vi "first_enable.vi"(2 "error out 2":errorcluster, 3 "VISA resource name 2":refnum<visa-resource-name>) -> (0 "error out 3":errorcluster, 1 "VISA resource name 3":refnum<visa-resource-name>)   [LabVIEW 2017]
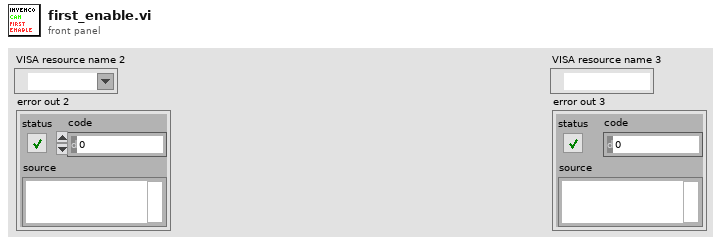
[diagram p1: front panel]
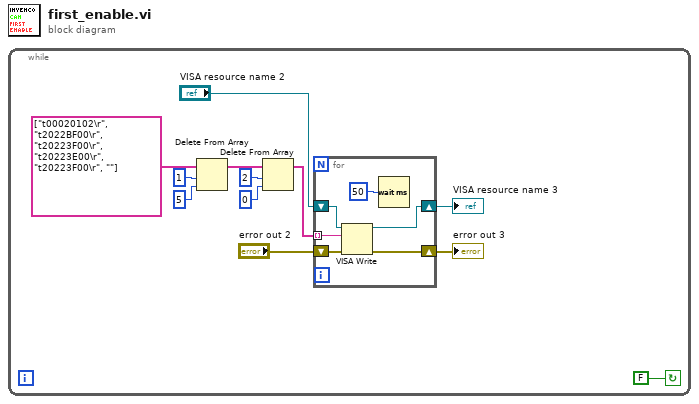
[diagram p0: block diagram]
diagram:
  n1 = while {
    stop <- FALSE continue-if-true
    n2 = Delete From Array(array=string[] ["t00020102\r", "t2022BF00\r", "t20223F00\r", "t20223E00\r", "t20223F00\r", ""], length=1, index=5) -> (array with subset deleted=w6:string[])  [unwired: 1 out]
    n3 = Delete From Array(array=w6, length=2, index=0) -> (array with subset deleted=w5:string[])  [unwired: 1 out]
    n4 = for {
      tunnel: w5 -> [w13] mode=indexing
      shift-right: [w16] -> w12
      shift-left: "VISA resource name 2" -> [w18]
      shift-right: [w15] -> w11
      shift-left: "error out 2" -> [w17]
      n5 = VISA Write(VISA resource name=w18, write buffer=w13, error in (no error)=w17) -> (VISA resource name out=w16:refnum<visa-resource-name>, error out=w15:errorcluster)  [unwired: 1 out]
      n6 = Wait (ms)(milliseconds to wait=u32 50 ("millisecond multiple")) -> ()  [unwired: 1 out]
    }
    "VISA resource name 3" <- w12
    "error out 3" <- w11
  }
